vi "Load Recipe from XML.vi"(8 "error in (no error)":errorcluster, 11 "Path":path) -> (0 "error out":errorcluster, 3 "Selected Recipe Settings":refnum<class "Process Settings.lvclass">)   [LabVIEW 2017, in "Process Settings.lvclass"]
uses:
  Process Settings.lvclass
  <vilib>/Utility/xml.llb/Read From XML File(string).vi
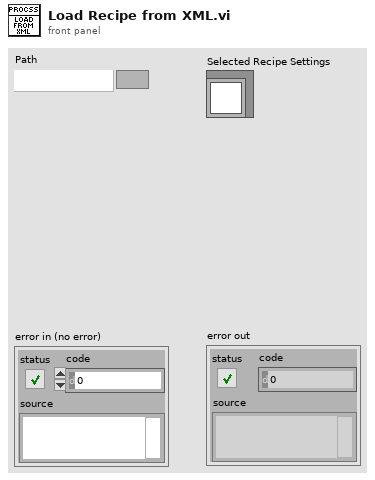
[diagram p1: front panel]
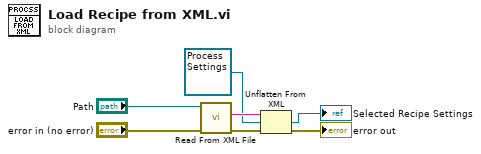
[diagram p0: block diagram]
diagram:
  n1 = call-poly <vilib>:"Read From XML File.vi"("error in (no error)"="error in (no error)", "XML File Path"="Path") -> ("error out"=w3:errorcluster, "XML Elements"=w5:string)  [unwired: 7 in, 1 out]
  n2 = Unflatten From XML(xml string=w5, type=refnum<class "Process Settings.lvclass"> refnum ("Process Settings.lvclass"), error in (no error)=w3) -> (value=→"Selected Recipe Settings":refnum<class "Process Settings.lvclass">, error out=→"error out":errorcluster)
